vi "GetClassName.vi"(0 "reference in":refnum<class "G#RemoteProxy.lvclass">, 5 "error in (no error)":errorcluster) -> (14 "reference out":refnum<class "G#RemoteProxy.lvclass">, 15 "class name":string, 16 "lvlib hierarchy":string[](array[string]), 17 "full class name":string, 19 "error out":errorcluster)   [LabVIEW 2017, in "G#RemoteProxy.lvclass"]
doc: "Returns the class name, full class name , lvlib hierarchy for the specified object."
uses:
  <vilib>/addons/_AddQ/G#Debugger/G#RemoteProxy/G#RemoteProxy.lvclass
  <vilib>/addons/_AddQ/G#Debugger/G#RemoteProxy/G#RemoteProxy.lvclass/G#RemoteProxy.ctl
  <vilib>/addons/_AddQ/G#Object/G#Object.lvclass
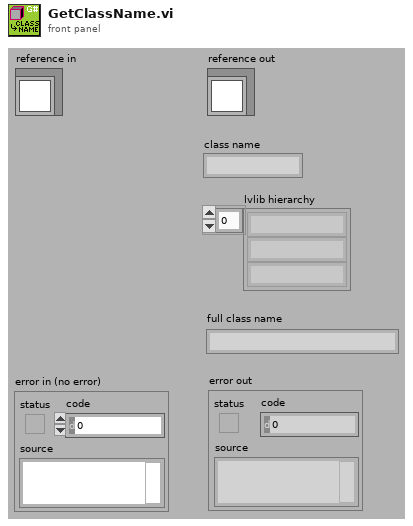
[diagram p1: front panel]
types:
  T1 = typedef "G#RemoteProxy.lvclass/ObjectAttributesProxy.ctl" = cluster{"class hierarchy":T2[], "class name":string, "lvlib hierarchy":string[], "full class name":string, "id":u32, "owner":string, "RemoteRef":refnum<class "G#Object.lvclass">, "object name":string, "attributes":variant[], "connection ID":refnum<k5>, "address":u32, "occurrence":refnum<k4>, "ProxyClassRef":refnum<class "G#RemoteProxy.lvclass">, "InMemory?":bool, "ToString":string}
  T2 = typedef "G#Object.lvclass/G#Object_ClassHierarchy.ctl" = cluster{"ClassName":string, "FullClassName":string, "ClassPath":path, "IsLeaf":bool}
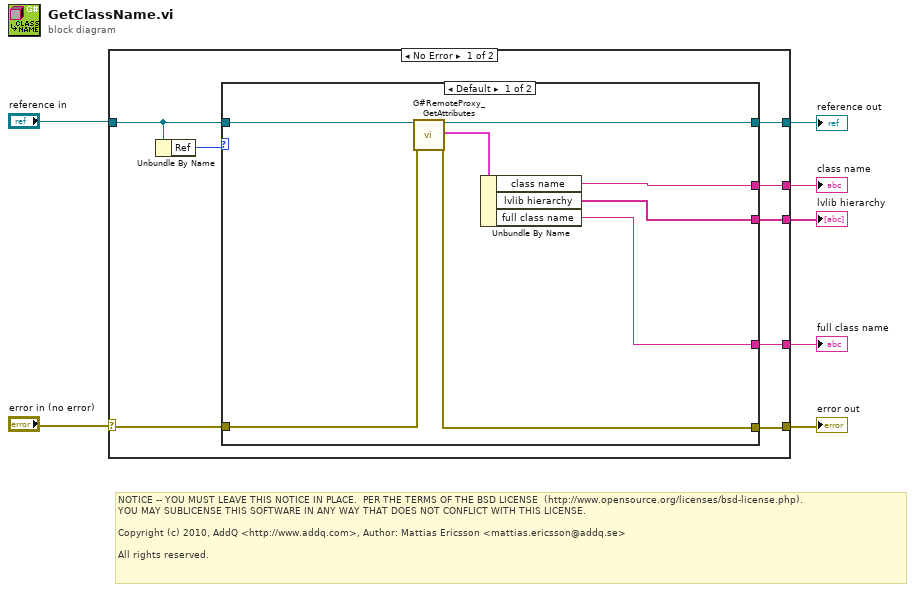
[diagram p0: block diagram]
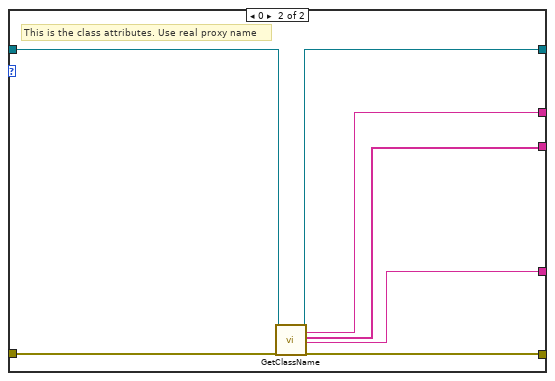
[diagram p2: hidden frame]
diagram:
  # "NOTICE -- YOU MUST LEAVE THIS NOTICE IN PLACE.  PER THE TERMS OF THE BSD LICENSE  (http://www.opensource.org/licenses/bsd-license.php).\nYOU MAY SUBLICENSE THIS SOFTWARE IN ANY WAY THAT DOES NOT CONFLICT WITH THIS LICENSE.\n\nCopyright (c) 2010, AddQ <http://www.addq.com>, Author: Mattias Ericsson <mattias.ericsson@addq.se>\n\nAll rights reserved."
  n1 = case shown="No Error" "error in (no error)" {
    selector: "error in (no error)" -> [w15 w31]
    tunnel: "reference in" -> [w9 w32]
    tunnel: [w14 w31] -> w1
    tunnel: [w13 w32] -> w6
    tunnel: [w12 _] -> w5
    tunnel: [w11 _] -> w4
    tunnel: [w10 _] -> w3
    frame No Error {
      n2 = Unbundle By Name(w9) -> ("Ref"=w8:u32)
      n3 = case shown="Default" w8 {
        tunnel: w15 -> [w23 w28]
        tunnel: [w22 w27] -> w14
        tunnel: [w21 w29] -> w13
        tunnel: [w19 w25] -> w12
        tunnel: [w16 w26] -> w11
        tunnel: [w18 w24] -> w10
        tunnel: w9 -> [w17 w30]
        frame Default {
          n4 = call <vilib>:"G#RemoteProxy_GetAttributes.vi"("reference in"=w17, "error in (no error)"=w23) -> ("reference out"=w21:refnum<class "G#RemoteProxy.lvclass">, "attributes"=w20:T1, "error out"=w22:errorcluster)  [unwired: 14 in, 1 out]
          n5 = Unbundle By Name(w20) -> ("class name"=w16:string, "lvlib hierarchy"=w19:string[], "full class name"=w18:string)
        }
        frame 0 {
          # "This is the class attributes. Use real proxy name"
          n6 = call-parent "GetClassName.vi"("reference in"=w30, "error in (no error)"=w28) -> ("reference out"=w29:refnum<class "G#RemoteProxy.lvclass">, "class name"=w26:string, "lvlib hierarchy"=w25:string[], "full class name"=w24:string, "error out"=w27:errorcluster)  [unwired: 13 in]
        }
      }
    }
    frame Error {
    }
  }
  "reference out" <- w6
  "class name" <- w4
  "lvlib hierarchy" <- w5
  "full class name" <- w3
  "error out" <- w1
